vi "SPA_Query.vi"(0 "System no.":i32=1 min=1 max=4 step=1, 2 "Axes to query":string[](array[string]), 3 "Parameter no.":i32[](array[numeric]), 4 "Without axes?":bool, 5 "error in":errorcluster, 6 "Parameter no. (hex)":u32[](array[numeric]) format="%.0x", 7 "Parameter no. format \n(Decimal: FALSE)":bool) -> (14 "Parameter value":dbl[](array[numeric]) format="%.6f", 15 "Parameter string":string[](array[string]), 16 "Queried axes out":string[](array[string]), 17 "Parameter no. out":i32[](array[numeric]), 18 "Parameter no. (hex) out":u32[](array[numeric]) format="%.0x", 19 "error out":errorcluster)   [LabVIEW 2020]
doc: "Returns parameter values for queried items and parameter numbers. For axis-related parameters, Axis to query is the axis name; for piezo-, sensor-, PIShift or demux-related parameters, the channel number, otherwise a parameter-related code. If parameter no. is in decimal format, use \"Parameter no.\" input, for hexadecimal parameter numbers use \"Parameter no. (hex)\" input and switch \"Parameter no. format\" to TRUE. If \"Without axes\" is TRUE, all available parameters for all axes/designators are returned. For parameter numbers which output a string use \"Parameter string\" output. See GCS DLL manual for available parameter numbers.\n\nC-413: Parameter no. format is TRUE (hex.). Use HPA?.vi to get valid parameter numbers. Do not query more than 6 parameter no. at once (except with Without axes? = TRUE).\n\nC-702: Parameter no. format is FALSE (decimal).\n\nC-843: Parameter no. format is FALSE (decimal). The following parameter number outputs a string:\n60: stage name (maximum 14 characters)\n\nC-843.PM: Parameter no. format is FALSE (decimal). The following parameter number outputs a string:\n60: stage name (maximum 14 characters)\n\nC-865: Parameter no. format is FALSE (decimal). The following parameter number outputs a string: 60: stage name (maximum 14 characters). Parameter number 25 is read-only.\n\nC-866: Parameter no. format is FALSE (decimal). The following parameter number outputs a string: 60: stage name (maximum 14 characters). Parameter number 25 is read-only.\n\nC-867, C-877: Parameter no. format is TRUE (hex.). Use HPA?.vi to get valid parameter numbers. Only one parameter value for only one axis per command allowed. Use \"Without axes?\" = TRUE for a query of all parameters.\n\nC-880: Parameter no. format is FALSE (decimal). Additional read-only parameter numbers are:\n- 14: Numerator of the counts per physical unit factor (1 to 2147483647) \n(factor = num./denom.))\n- 15: Denominator of the counts per physical unit factor (1 to 2147483647) \n(factor = num./denom.)\n- 16: Drive mode: 0=Analog 1=PWM\n- 19: Axis type: 0=Linear 1=Rotary\n- 20: Reference switch: 0=no present, 1=present\n- 28: Reference status: 0=axis not referenced; 1=axis is referenced\n\nC-880K005: VI only supported when called through PI_Multix.vi\n\nC-884: Parameter no. format is TRUE (hex.). Use HPA?.vi to get valid parameter numbers. Do not query more than 4 parameter no. at once (except with Without axes? = TRUE) Use Without axes? = TRUE for a query of all parameters.\n\nC-891: Parameter no. format is TRUE (hex.). Use HPA?.vi to get valid parameter numbers. Do not query more than 1 parameter no. at once (except with Without axes? = TRUE).\n\nE-135: Parameter no. format is TRUE (hex.). Use HPA?.vi to get valid parameter numbers.\n\nE-516: Parameter no. format is FALSE (decimal).\n\nE-517, E-518: Parameter no. format is TRUE (hex.). Use HPA?.vi to get valid parameter numbers.\n\nE-709: Parameter no. format is TRUE (hex.). Only one parameter value for only one axis per command allowed. Use Without axes? = TRUE for a query of all parameters. Use HPA?.vi to get valid parameter numbers. \n\nE-710: Use HPA?.vi to get valid parameter numbers and see GCS DLL manual for a description of valid parameter numbers. Parameter no. format is TRUE (Hex).\n\nE-712: Parameter no. format is TRUE (hex.). Use HPA?.vi to get valid parameter numbers. Do not query more than 10 parameter no. at once (except with \"Without axes? = TRUE).\n\nE-725, E-727: Parameter no. format is TRUE (hex.). Use HPA?.vi to get valid parameter numbers. Do not query more than 10 parameter no. at once (except with Without axes? = TRUE).\n\nE-753: Parameter no. format is TRUE (hex.). Use HPA?.vi to get valid parameter numbers.\n\nE-754: Parameter no. format is TRUE (hex.). Use HPA?.vi to get valid parameter numbers.\n\nE-755: Parameter no. format is TRUE (hex.). Use HPA?.vi to get valid parameter numbers. \n\nE-761: Use HPA?.vi to get valid parameter numbers and see GCS DLL manual for a description of valid parameter numbers. Parameter no. format is TRUE (Hex). Do not query more than 10 parameter no. at once (except with Without axes? = TRUE).\n\nE-816: Parameter no. format is FALSE (decimal). Only one parameter value for only one axis per command allowed. This command cannot be issued to a slave\n\nE-861: Parameter no. format is TRUE (hex.). Use HPA?.vi to get valid parameter numbers. Only one parameter value for only one axis per command allowed. Use \"Without axes?\" = TRUE for a query of all parameters. The following parameter number outputs a string:\n60 (0x3C): stage name (maximum 16 characters)\n\nE-870: Parameter no. format is TRUE (hex.). Use HPA?.vi to get valid parameter numbers. Only one parameter value for only one channel per command allowed. Use Without axes? = TRUE for a query of all parameters.\n\nE-871, E-872, E-873, E-874: Parameter no. format is TRUE (hex.). Use HPA?.vi to get valid parameter numbers. Only one parameter value for only one axis per command allowed. Use Without axes? = TRUE for a query of all parameters.\n\nC-887, F-206: Only for GCS syntax version = GCS 2.0 or higher (Check with CSV?.vi. If CSV?.vi is not supported, syntax version is GCS 1.0). Parameter no. format is TRUE (hex.). Use HPA?.vi to get valid parameter numbers. Length of command is limited by firmware (appr. 10 parameters per call), see controller user manual for details. Use Without axes? = TRUE for a query of all parameters.\n\nHydra, Pollux: Parameter no. format is TRUE (hex.). Use HPA?.vi to get valid parameter numbers. Do not query more than 10 parameter no. at once (except with Without axes? = TRUE) Use Without axes? = TRUE for a query of all parameters.\n\nC-887, M-8X0: \nFor GCS syntax version = GCS 2.0 or higher (Check with CSV?.vi. If CSV?.vi is not supported, syntax version is GCS 1.0), Parameter no. format is TRUE (hex.). Use HPA?.vi to get valid parameter numbers. Length of command is limited by firmware (appr. 10 parameters per call), see controller user manual for details. Use Without axes? = TRUE for a query of all parameters.\nFor GCS syntax version = GCS 1.0, Parameter no. format is FALSE (decimal), Axes to query can be 1 to 6 (corresponds to strut no.) and Parameter no. can be 512 (reports if strut is extended or retracted) or 513 (reports commanded strut length). Only one parameter value for only one axis per command allowed.\n\nMercury: Parameter no. format is FALSE (decimal). The following parameter number outputs a string: 60: stage name (maximum 14 characters)\n\nMercury_GCS: Parameter no. format is TRUE (hex.). Use HPA?.vi to get valid parameter numbers. Only one parameter value for only one axis per command allowed. Use Without axes? = TRUE for a query of all parameters."
uses:
  Global1.vi
panel:
  # "Returns parameter values for queried items and parameter numbers. If parameter no. is in decimal format, use \"Parameter no.\" \ninput, for hexadecimal parameter numbers use \"Parameter no. (hex)\" input and switch \"Parameter no. format\" to TRUE. For para-\nmeter numbers which output a string use \"Parameter string\" output."
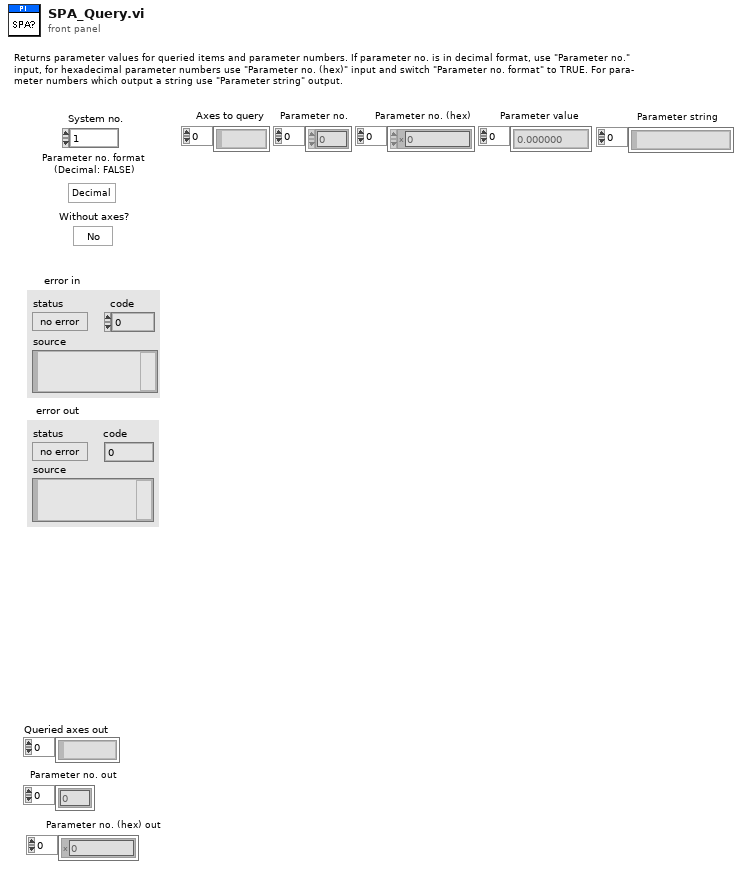
[diagram p1: front panel]
types:
  T1 = enum16{"Disable error check", "Force error check", "Use global settings"}
  T2 = typedef "Syntax.ctl" = enum16{"GCS 1.0", "GCS 2.0", "GCS 3.0"}
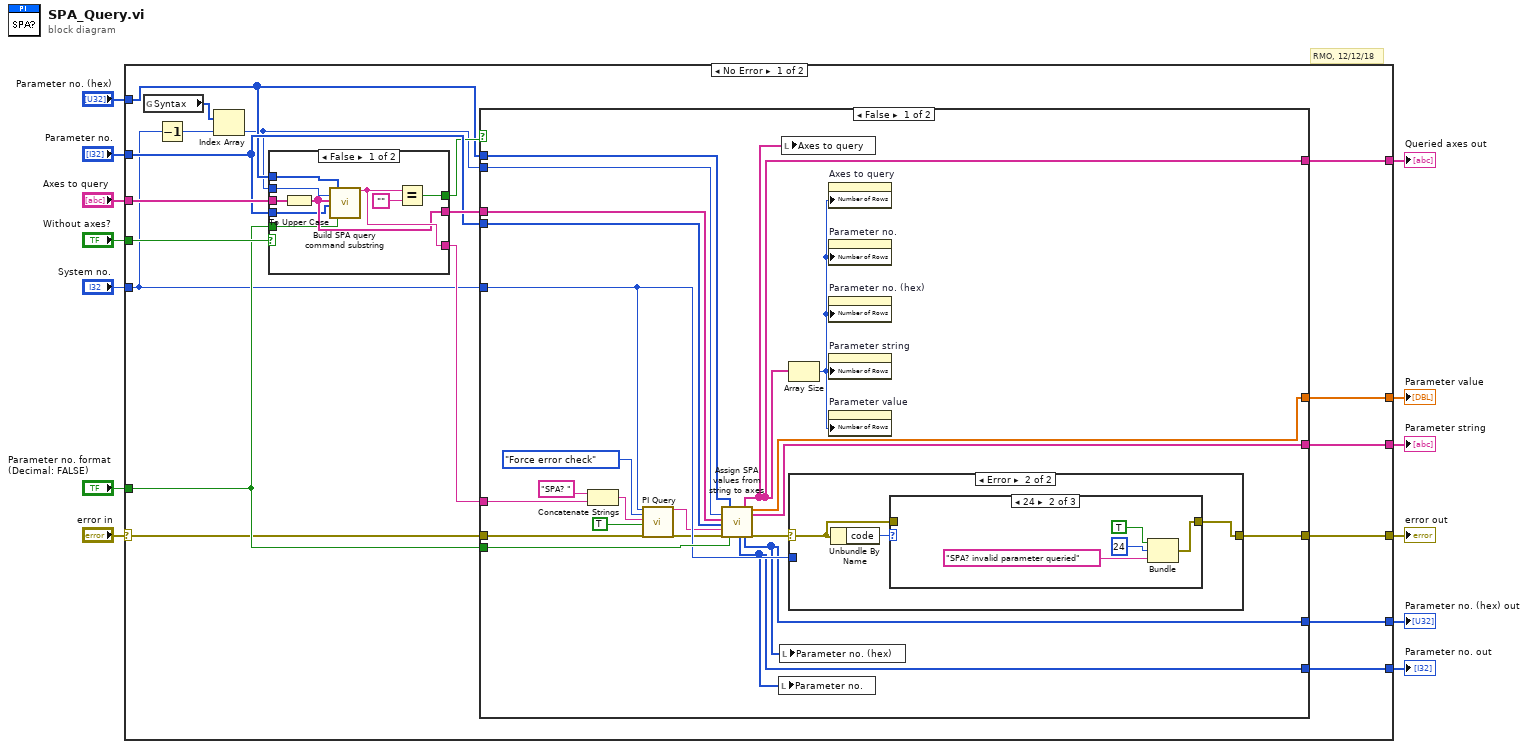
[diagram p0: block diagram]
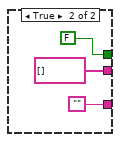
[diagram p2: hidden frame]
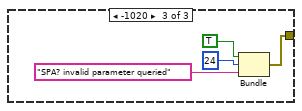
[diagram p5: hidden frame]
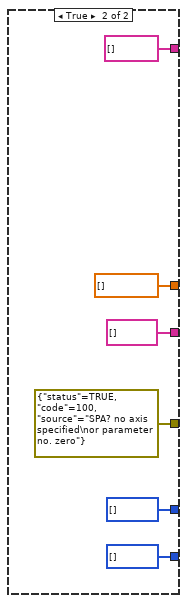
[diagram p6: hidden frame]
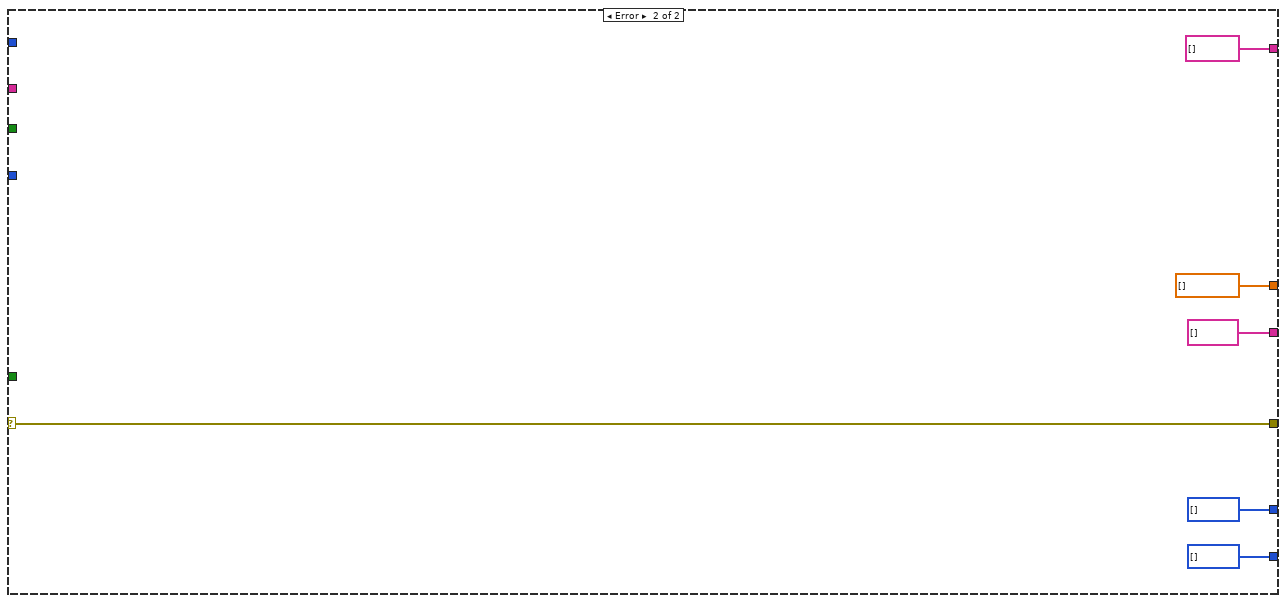
[diagram p7: hidden frame]
diagram:
  # "RMO, 12/12/18"
  n1 = case shown="No Error" "error in" {
    selector: "error in" -> [w14 w86]
    tunnel: "Axes to query" -> [w32 _]
    tunnel: "System no." -> [w19 _]
    tunnel: "Parameter no." -> [w29 _]
    tunnel: [w28 w86] -> w10
    tunnel: [w26 dbl[] [] ("Parameter values")] -> w9
    tunnel: "Parameter no. (hex)" -> [w24 _]
    tunnel: "Parameter no. format \n(Decimal: FALSE)" -> [w23 _]
    tunnel: "Without axes?" -> [w25 _]
    tunnel: [w22 string[] [] ("Parameter strings")] -> w5
    tunnel: [w17 string[] [] ("Queried axes out")] -> w4
    tunnel: [w16 i32[] [] ("Parameter no. out")] -> w3
    tunnel: [w15 u32[] [] ("Parameter no. (hex) out")] -> w2
    frame No Error {
      n2 = global read "Global1.vi" "Syntax"() -> (w20:T2[])
      n3 = Decrement(x=w19) -> (x-1=w21:i32)
      n4 = Index Array(array=w20, index=w21) -> (element=w18:T2)
      n5 = case shown="False" w25 {
        tunnel: w32 -> [w41 _]
        tunnel: [w40 "" ("Command substring")] -> w31
        tunnel: [w39 string[] [] ("Designator to query")] -> w30
        tunnel: w29 -> [w38 _]
        tunnel: [w37 FALSE] -> w27
        tunnel: w24 -> [w36 _]
        tunnel: w23 -> [w35 _]
        tunnel: w18 -> [w34 _]
        frame False {
          n6 = To Upper Case(1:w41) -> (0:w39:string[])
          n7 = call "Build SPA query command substring.vi"("Syntax"=w34, "Axes to query"=w39, "Parameter number"=w38, "Parameter number (hex)"=w36, "Parameter no. format \n(Decimal: FALSE)"=w35) -> ("Command substring"=w40:string)  [unwired: 2 in, 12 out]
          n8 = Equal?(x=w40, y="" ("x")) -> (x = y?=w37:bool)
        }
        frame True {
        }
      }
      n9 = case shown="False" w27 {
        tunnel: w14 -> [w57 _]
        tunnel: w31 -> [w63 _]
        tunnel: w30 -> [w62 _]
        tunnel: w19 -> [w54 _]
        tunnel: w29 -> [w61 _]
        tunnel: [w59 errorcluster {"status"=TRUE, "code"=100, "source"="SPA? no axis specified\nor parameter no. zero"} ("error out")] -> w28
        tunnel: [w60 dbl[] [] ("Parameter values")] -> w26
        tunnel: w24 -> [w55 _]
        tunnel: w23 -> [w56 _]
        tunnel: [w58 string[] [] ("Parameter strings")] -> w22
        tunnel: w18 -> [w53 _]
        tunnel: [w50 string[] [] ("Queried axes out")] -> w17
        tunnel: [w52 i32[] [] ("Parameter no. out")] -> w16
        tunnel: [w51 u32[] [] ("Parameter no. (hex) out")] -> w15
        frame False {
          n10 = Concatenate Strings("SPA? ", w63) -> (w64:string)
          n11 = call "PI Query.vi"("System no."=w54, "Error check settings"=T1."Force error check", "String to send"=w64, "Attach termination char.?"=TRUE ("Attach Linefeed?"), "error in"=w57) -> ("String read"=w48:string, "error out"=w47:errorcluster)  [unwired: 2 in, 11 out]
          n12 = call "Assign SPA values from string to axes.vi"("Syntax"=w53, "Queried axes"=w62, "Parameter no."=w61, "Input string"=w48, "error in"=w47, "Parameter no. (hex)"=w55, "Parameter no. format \n(Decimal: FALSE)"=w56) -> ("Parameter no. out"=w52:i32[], "Queried axes out"=w50:string[], "Parameter no. (hex) out"=w51:u32[], "Parameter values"=w60:dbl[], "Parameter strings"=w58:string[], "error out"=w46:errorcluster)  [unwired: 1 in, 6 out]
          n13 = local write "Parameter no."(w52) -> ()
          n14 = local write "Parameter no. (hex)"(w51) -> ()
          n15 = local write "Axes to query"(w50) -> ()
          n16 = Array Size(array=w50) -> (size(s)=w49:i32)
          n17 = case shown="Error" w46 {
            selector: w46 -> [w67 w69]
            tunnel: [w67 w70] -> w59
            tunnel: w54 -> [_ _]
            frame No Error {
            }
            frame Error {
              n18 = Unbundle By Name(w69) -> ("code"=w68:i32)
              n19 = case shown="24" w68 {
                tunnel: [w71 w72 w76] -> w70
                tunnel: w69 -> [w71 _ _]
                frame 0, Default {
                }
                frame 24 {
                  n20 = Bundle(TRUE, 24, "SPA? invalid parameter queried") -> (w72:errorcluster)  [unwired: 1 out]
                }
                frame -1020 {
                  n21 = Bundle(TRUE, 24, "SPA? invalid parameter queried") -> (w76:errorcluster)  [unwired: 1 out]
                }
              }
            }
          }
          n22 = property on="Axes to query" class="Arr (strict)"("Number of Rows"=w49) -> ()  [unwired: 2 in, 2 out]
          n23 = property on="Parameter no." class="Arr (strict)"("Number of Rows"=w49) -> ()  [unwired: 2 in, 2 out]
          n24 = property on="Parameter no. (hex)" class="Arr (strict)"("Number of Rows"=w49) -> ()  [unwired: 2 in, 2 out]
          n25 = property on="Parameter string" class="Arr (strict)"("Number of Rows"=w49) -> ()  [unwired: 2 in, 2 out]
          n26 = property on="Parameter value" class="Arr (strict)"("Number of Rows"=w49) -> ()  [unwired: 2 in, 2 out]
        }
        frame True {
        }
      }
    }
    frame Error {
    }
  }
  "error out" <- w10
  "Parameter value" <- w9
  "Parameter string" <- w5
  "Queried axes out" <- w4
  "Parameter no. out" <- w3
  "Parameter no. (hex) out" <- w2
